vi "Actor Core.vi"(8 "error in":errorcluster, 11 "Sequencer in":refnum<class "Sequencer.lvclass">) -> (0 "error out":errorcluster, 3 "Actor out":refnum<class "Actor.lvclass">)   [LabVIEW 2020, in "Sequencer.lvlib" / "Sequencer.lvclass"]
doc: "(<B>Filename</B>: Actor Framework.lvlib:Actor.lvclass:Actor Core.vi)\n\nReceives messages to the actor, reacts to them, and initiates any error handling that may shut the actor down.\n\nDescendant classes may override this VI to append parallel tasks for the actor to complete while it handles messages. Overrides use the Call Parent Method node.\n\nThis implementation runs a Sequencer Core in parallel to the Actor Core."
uses:
  Sequencer.lvclass
  C:/Current projects/WS/PPL/HDH.Actor Framework.Core.Actor.lvlibp/1abvi3w/vi.lib/ActorFramework/Actor/Actor.lvclass
  PPL/HDH.Actor Framework.Core.Actor.lvlibp/1abvi3w/vi.lib/ActorFramework/Actor/Actor.lvclass
  Sequencer.lvclass/Sequencer.ctl
  Sequencer Core/Sequencer Core.lvclass/Sequencer Core.ctl
  Sequencer Messages/Terminate Sequncer Msg/Terminate Sequencer Msg.lvclass
  PPL/HDH.Actor Framework.Core.Actor.lvlibp/1abvi3w/vi.lib/ActorFramework/Message Enqueuer/Message Priority.ctl
  PPL/HDH.Actor Framework.Core.Actor.lvlibp/1abvi3w/vi.lib/ActorFramework/Message/Message.lvclass
  Sequencer Core/Sequencer Core.lvclass
  PPL/HDH.Actor Framework.Core.Actor.lvlibp/1abvi3w/vi.lib/ActorFramework/Message Enqueuer/Message Enqueuer.lvclass
  C:/Current projects/WS/PPL/HDH.Actor Framework.Core.Actor.lvlibp/1abvi3w/vi.lib/ActorFramework/Message/Message.lvclass
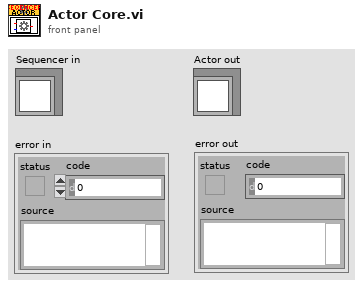
[diagram p1: front panel]
types:
  T1 = typedef "HDH.Actor Framework.Core.Actor.lvlibp/Message Enqueuer.lvclass/Message Priority.ctl" = enum16{"Low", "Normal", "High"}
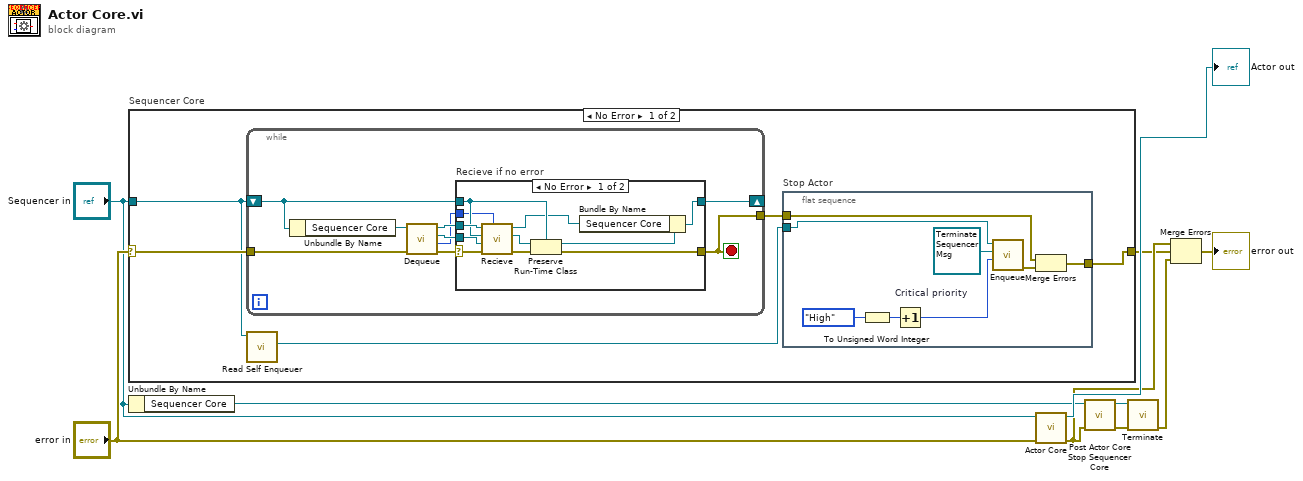
[diagram p0: block diagram]
diagram:
  n1 = case "Sequencer Core" shown="No Error" "error in" {
    selector: "error in" -> [w15 w46]
    tunnel: "Sequencer in" -> [w14 _]
    tunnel: [w12 w46] -> w2
    frame No Error {
      n2 = while {
        tunnel: [w30] -> w11
        tunnel: w15 -> [w29]
        shift-right: [w25] -> _
        shift-left: w14 -> [w24]
        stop <- w30 stop-if-true
        n3 = Unbundle By Name(w24) -> ("Sequencer Core"=w32:refnum<class "Sequencer Core.lvclass">)
        n4 = call "Dequeue.vi"("error in (no error)"=w29, "Sequencer Core in"=w32) -> ("error out"=w31:errorcluster, "Message Priority"=w26:T1, "Message"=w27:refnum<class "Message.lvclass">, "Sequencer Core out"=w28:refnum<class "Sequencer Core.lvclass">)  [unwired: 6 in]
        n5 = case "Recieve if no error" shown="No Error" w31 {
          selector: w31 -> [w39 w45]
          tunnel: [w37 w45] -> w30
          tunnel: w28 -> [w43 _]
          tunnel: w27 -> [w35 _]
          tunnel: w26 -> [w36 _]
          tunnel: [w34 w44] -> w25
          tunnel: w24 -> [w42 w44]
          frame No Error {
            n6 = call "Recieve.vi"("Message Priority"=w36, "error in (no error)"=w39, "Message"=w35, "Actor in"=w42, "Sequencer Core in"=w43) -> ("error out"=w38:errorcluster, "Actor out"=w41:refnum<class "Actor.lvclass">, "Sequencer Core out"=w33:refnum<class "Sequencer Core.lvclass">)  [unwired: 4 in]
            n7 = Preserve Run-Time Class(object in=w41, error in=w38, 2:w42) -> (object out=w40:refnum<class "Sequencer.lvclass">, error out=w37:errorcluster)
            n8 = Bundle By Name(cluster=w40, "Sequencer Core"=w33) -> (w34:refnum<class "Sequencer.lvclass">)
          }
          frame Error {
          }
        }
      }
      n9 = call "Read Self Enqueuer.vi"("Actor"=w14) -> ("Self Enqueuer"=w13:refnum<class "Message Enqueuer.lvclass">)  [unwired: 10 in]
      n10 = flat-sequence "Stop Actor" {
        tunnel: w13 -> [w21]
        tunnel: [w23] -> w12
        tunnel: w11 -> [w22]
        frame #0 {
          n11 = To Unsigned Word Integer(number=Message_Priority."High" ("Message Priority (Normal)")) -> (unsigned 16bit integer=w16:u16)
          n12 = Increment "Critical priority"(x=w16) -> (x+1=w18:u16)
          n13 = call "Enqueue.vi"("Message Priority (Normal)"=w18, "Message"=refnum<class "Terminate Sequencer Msg.lvclass"> refnum ("Sequencer.lvlib:Terminate Sequncer Msg.lvclass"), "Message Enqueuer in"=w21) -> ("error out"=w17:errorcluster)  [unwired: 7 in, 1 out]
          n14 = Merge Errors(w22, w17) -> (w23:errorcluster)
        }
      }
    }
    frame Error {
    }
  }
  n15 = Unbundle By Name("Sequencer in") -> ("Sequencer Core"=w6:refnum<class "Sequencer Core.lvclass">)
  n16 = call-parent "Actor Core.vi"("error in"="error in", "Actor in"="Sequencer in") -> ("error out"=w3:errorcluster, "Actor out"=→"Actor out":refnum<class "Actor.lvclass">)  [unwired: 8 in]
  n17 = call "Post Actor Core Stop Sequencer Core.vi"("error in (no error)"=w3, "Sequencer Core in"=w6) -> ("error out"=w5:errorcluster, "Sequencer Core out"=w4:refnum<class "Sequencer Core.lvclass">)  [unwired: 8 in]
  n18 = call "Terminate.vi"("error in (no error)"=w5, "Sequencer Core in"=w4) -> ("error out"=w1:errorcluster)  [unwired: 8 in, 1 out]
  n19 = Merge Errors(w3, w2, w1) -> (→"error out":errorcluster)
